vi "WriteToFile.vi"(8 "error in":errorcluster, 10 "LastAccess Time":i32, 11 "Elapse Time":i32) -> (0 "error out":errorcluster)   [LabVIEW 2021]
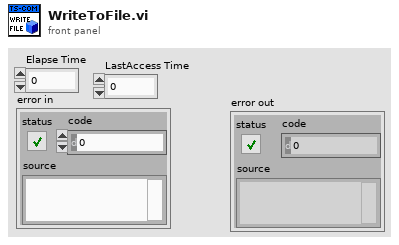
[diagram p1: front panel]
types:
  T1 = enum16{"open", "replace", "create", "open or create", "replace or create", "replace or create with confirmation"}
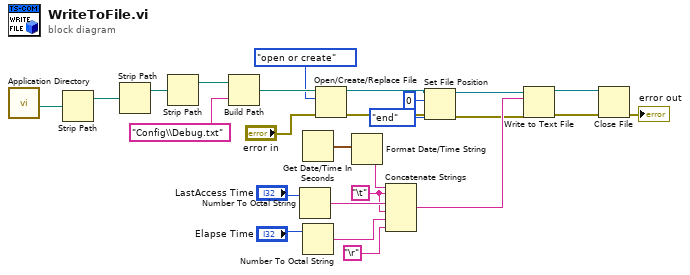
[diagram p0: block diagram]
diagram:
  w1 = "\t"
  n1 = call <vilib>:"Application Directory.vi"() -> ("Application Directory"=w22:path)
  n2 = Strip Path(path=w22) -> (stripped path=w23:path)  [unwired: 1 out]
  n3 = Strip Path(path=w23) -> (stripped path=w25:path)  [unwired: 1 out]
  n4 = Strip Path(path=w25) -> (stripped path=w26:path)  [unwired: 1 out]
  n5 = Build Path(base path=w26, name or relative path="Config\\Debug.txt") -> (appended path=w21:path)
  n6 = Number To Octal String(2:"LastAccess Time") -> (0:w6:string)  [unwired: 1 in]
  n7 = Get Date/Time In Seconds() -> (seconds since 1Jan1904=w8:timestamp)
  n8 = Number To Octal String(2:"Elapse Time") -> (0:w3:string)  [unwired: 1 in]
  n9 = Open/Create/Replace File(file path (use dialog)=w21, error in="error in", operation (0:open)=T1."open or create") -> (refnum out=w12:refnum<file>, error out=w14:errorcluster)  [unwired: 3 in, 1 out]
  n10 = Format Date/Time String(seconds (now)=w8) -> (date/time string=w7:string)  [unwired: 2 in]
  n11 = Concatenate Strings(w7, w1, w6, w1, w3, "\r") -> (w15:string)
  n12 = Set File Position(offset (in bytes) (0)=i64 0, refnum=w12, from (0:start)=enum16{"start", "end", "current"}."end", error in=w14) -> (refnum out=w11:refnum<file>, error out=w13:errorcluster)
  n13 = Write to Text File(file (use dialog)=w11, text=w15, error in=w13) -> (refnum out=w18:refnum<file>, error out=w19:errorcluster)  [unwired: 1 in, 1 out]
  n14 = Close File(refnum=w18, error in=w19) -> (error out=→"error out":errorcluster)  [unwired: 1 out]
